vi "DrawScreen.vi"(8 "error in (no error)":errorcluster, 11 "AttractScreen in":refnum<class "AttractScreen.lvclass">) -> (0 "error out":errorcluster, 3 "AttractScreen out":refnum<class "AttractScreen.lvclass">)   [LabVIEW 2019, in "RT_Game.lvlib" / "AttractScreen.lvclass"]
uses:
  AttractScreen.lvclass
  AttractStates.ctl
  AttractScreen.lvclass/AttractScreen.ctl
  Engine/Engine.lvclass
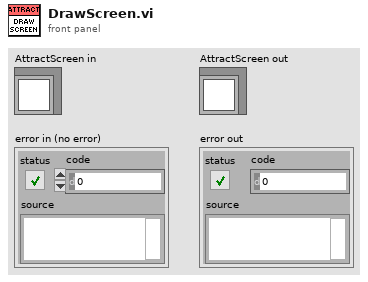
[diagram p1: front panel]
types:
  T1 = typedef "RT_Game.lvlib/AttractScreen.lvclass/AttractStates.ctl" = enum16{"FadeIn", "Display", "FadeOut"}
  T2 = typedef "RT_Game.lvlib/Engine.lvclass/TileCoordinate.ctl" = cluster{"x":i16, "y":i16}
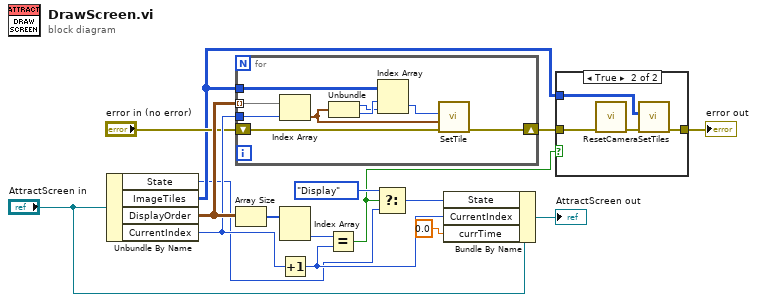
[diagram p0: block diagram]
diagram:
  n1 = Unbundle By Name("AttractScreen in") -> ("State"=w4:T1, "ImageTiles"=w7:u32[][], "DisplayOrder"=w15:T2[][], "CurrentIndex"=w13:i16)
  n2 = for {
    tunnel: w15 -> [w25] mode=indexing
    tunnel: w13 -> [w24]
    tunnel: w7 -> [w17]
    shift-right: [w19] -> w10
    shift-left: "error in (no error)" -> [w18]
    n3 = Index Array(array=w25, index=w24) -> (element=w23:T2)
    n4 = Unbundle(w23) -> ("x"=w20:i16, "y"=w21:i16)
    n5 = Index Array(array=w17, index (row)=w21, index (col)=w20) -> (element=w22:u32)
    n6 = call "SetTile.vi"("error in (no error)"=w18, "Coordinates"=w23, "TileCode"=w22) -> ("error out"=w19:errorcluster)  [unwired: 8 in]
  }
  n7 = Array Size(array=w15) -> (size(s)=w16:i32[])
  n8 = Index Array(array=w16) -> (element #2=w1:i32)  [unwired: 2 in, 1 out]
  n9 = Increment(x=w13) -> (x+1=w14:i16)
  n10 = Equal?(x=w1, y=w14) -> (x = y?=w3:bool)
  n11 = Select(t=AttractStates."Display" ("State"), s=w3, f=w4) -> (s? t:f=w5:T1)
  n12 = Bundle By Name(cluster="AttractScreen in", "State"=w5, "CurrentIndex"=w14, "currTime"=0.0) -> (→"AttractScreen out":refnum<class "AttractScreen.lvclass">)
  n13 = case shown="True" w3 {
    tunnel: w10 -> [w26 w30]
    tunnel: [w26 w29] -> w8
    tunnel: w7 -> [_ w28]
    frame False {
    }
    frame True {
      n14 = call "ResetCamera.vi"("error in (no error)"=w30) -> ("error out"=w27:errorcluster)  [unwired: 10 in]
      n15 = call "SetTiles.vi"("error in (no error)"=w27, "TileCodes"=w28) -> ("error out"=w29:errorcluster)  [unwired: 9 in]
    }
  }
  "error out" <- w8
